vi "sendAndWaitForResponse.vi"(6 "command to wait for (optional)":string, 8 "error in":errorcluster, 9 "read timeout":u32=4000, 10 "Command":string="Test", 11 "NetworkConnection in":refnum<class "NetworkConnection.lvclass">) -> (0 "error out":errorcluster, 1 "Read Cycles":i32, 2 "Msg Id":i32, 3 "NetworkConnection out":refnum<class "NetworkConnection.lvclass">, 4 "Messages":T1[](array[typedef]))   [LabVIEW 2020]
doc: "Provides a basic example of an RT user interface that uses network streams to connect to a PC.JKI Network Streams Connection 1.1.1.15\nJavier Ruiz - JKI\nCopyright (c) 2020, JKI\n\nThis library is provided \"AS IS\" ,WITHOUT WARRANTIES OR CONDITIONS OF ANY KIND, either express or implied."
uses:
  NetworkConnection.lvclass
  PublicSettings.ctl
  NetworkCommand--Cluster.ctl
  MGI Wait (U32).vi
panel:
  out "Timed Out?":bool
  out "StillConnected?":bool
  out "Public Settings":T2
  in  "Settings":T2
  out "Connected?":bool
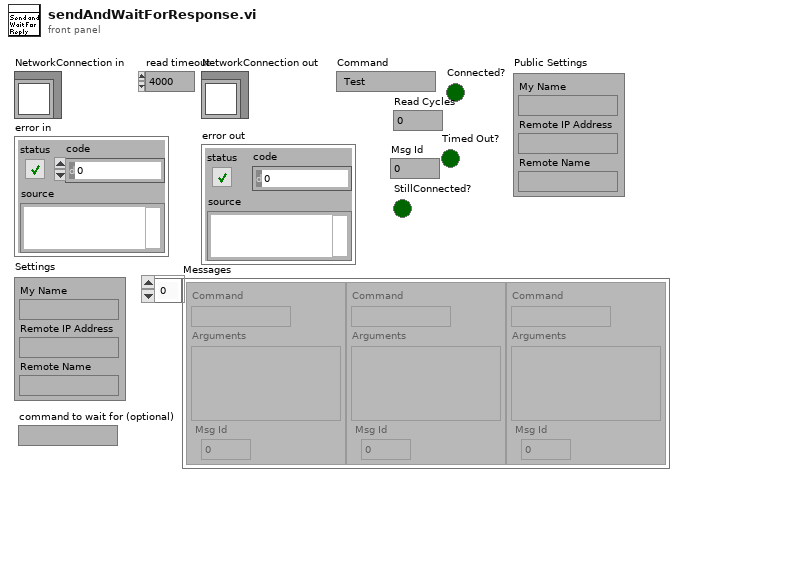
[diagram p1: front panel]
types:
  T1 = typedef "NetworkConnection.lvclass/NetworkCommand--Cluster.ctl" = cluster{"Command":string, "Arguments":variant, " Msg Id":i32}
  T2 = typedef "NetworkConnection.lvclass/PublicSettings.ctl" = cluster{"My Name":string, "Remote IP Address":string, "Remote Name":string}
  T3 = cluster{"Messages[0]":T1, "Messages[1]":T1, "Messages[2]":T1, "Messages[3]":T1, "Messages[4]":T1, "Messages[5]":T1, "Messages[6]":T1, "Messages[7]":T1, "Messages[8]":T1}
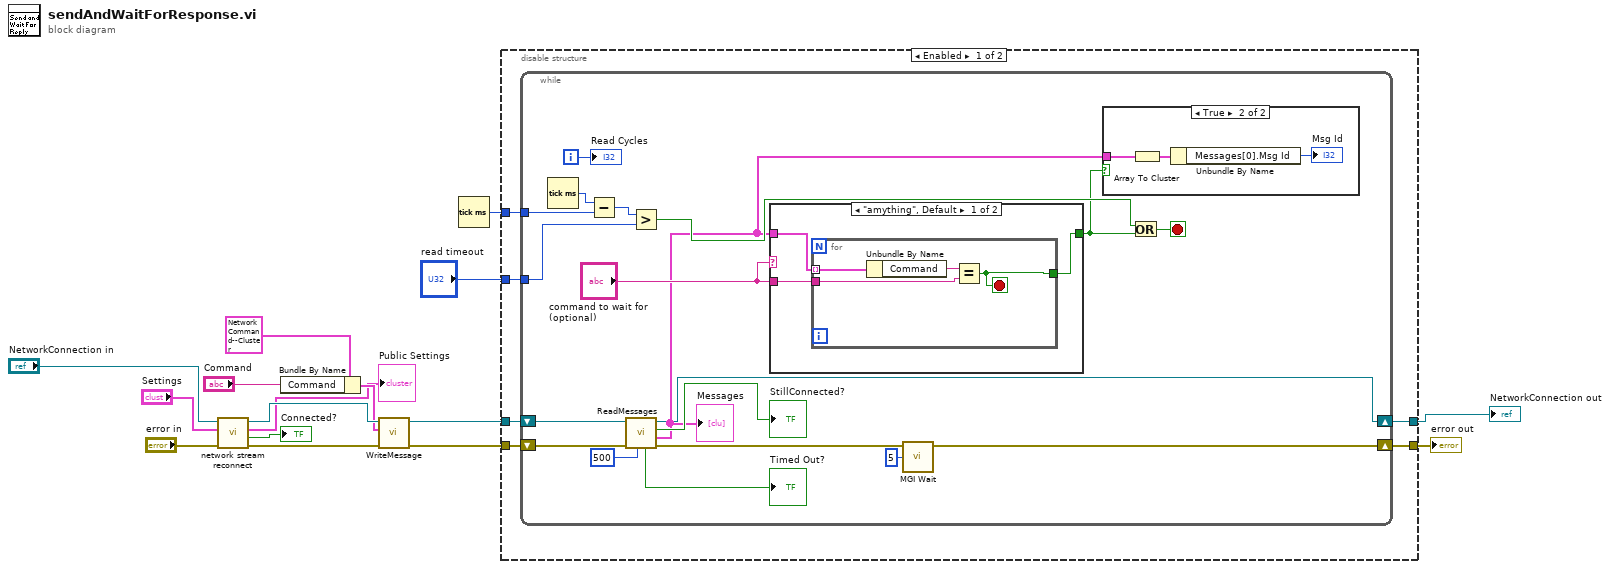
[diagram p0: block diagram]
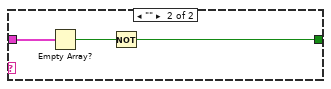
[diagram p2: hidden frame]
diagram:
  n1 = call "network stream reconnect.vi"("error in (no error)"="error in", "Settings"="Settings", "NetworkConnection in"="NetworkConnection in") -> ("error out"=w16:errorcluster, "Connected?"=→"Connected?":bool, "Public Settings"=→"Public Settings":T2, "NetworkConnection out"=w15:refnum<class "NetworkConnection.lvclass">)  [unwired: 5 in]
  n2 = Bundle By Name(cluster=T1 {"Command"="", "Arguments"=variant, " Msg Id"=0} ("Message"), "Command"="Command") -> (w9:T1)
  n3 = call "WriteMessage.vi"("error in (no error)"=w16, "Message"=w9, "NetworkConnection in"=w15) -> ("error out"=w13:errorcluster, "NetworkConnection out"=w14:refnum<class "NetworkConnection.lvclass">)  [unwired: 5 in, 2 out]
  n4 = Tick Count (ms)() -> (millisecond timer value=w2:u32)
  n5 = disable-structure shown="Enabled" {
    disable-tunnel: w14 -> [w22 w56]
    disable-tunnel: w13 -> [w21 w55]
    disable-tunnel: [w20 w56] -> w12
    disable-tunnel: [w19 w55] -> w11
    disable-tunnel: w2 -> [w18 _]
    disable-tunnel: "read timeout" -> [w17 _]
    frame Enabled {
      n6 = while {
        shift-right: [w41] -> w20
        shift-left: w22 -> [w39]
        shift-right: [w33] -> w19
        shift-left: w21 -> [w38]
        tunnel: w18 -> [w31]
        tunnel: w17 -> [w26]
        i -> [w37]
        stop <- w40 stop-if-true
        n7 = Tick Count (ms)() -> (millisecond timer value=w30:u32)
        n8 = Subtract(x=w30, y=w31) -> (x-y=w29:u32)
        n9 = call "ReadMessages.vi"("Timeout(ms)"=500, "error in (no error)"=w38, "NetworkConnection in"=w39) -> ("error out"=w34:errorcluster, "Messages"=w24:T1[], "StillConnected?"=→"StillConnected?":bool, "NetworkConnection out"=w41:refnum<class "NetworkConnection.lvclass">, "Timed Out?"=→"Timed Out?":bool)  [unwired: 4 in]
        "Messages" <- w24
        n10 = Greater?(x=w29, y=w26) -> (0:w36:bool)
        n11 = case shown="\"amything\", Default" "command to wait for (optional)" {
          tunnel: w24 -> [w44 w50]
          tunnel: "command to wait for (optional)" -> [w43 _]
          tunnel: [w42 w49] -> w23
          frame "amything", Default {
            n12 = for {
              tunnel: w44 -> [w48] mode=indexing
              tunnel: w43 -> [w46]
              tunnel: [w45] -> w42
              stop <- w45 stop-if-true
              n13 = Unbundle By Name(w48) -> ("Command"=w47:string)
              n14 = Equal?(x=w47, y=w46) -> (x = y?=w45:bool)
            }
          }
          frame "" {
            n15 = Empty Array?(array=w50) -> (empty?=w51:bool)
            n16 = Not(x=w51) -> (.not. x?=w49:bool)
          }
        }
        n17 = call-poly "MGI Wait.vi"("ms"=u32 5, "Error In"=w34) -> ("Error Out"=w33:errorcluster)  [unwired: 5 in]
        n18 = case shown="True" w23 {
          tunnel: w24 -> [_ w54]
          frame False {
          }
          frame True {
            n19 = Array To Cluster(array=w54) -> (cluster=w53:T3)
            n20 = Unbundle By Name(w53) -> ("Messages[0].Msg Id"=→"Msg Id":i32)
          }
        }
        n21 = Or(x=w36, y=w23) -> (x .or. y?=w40:bool)
        "Read Cycles" <- w37
      }
    }
    frame Disabled {
    }
  }
  "NetworkConnection out" <- w12
  "error out" <- w11
